vi "MCL Single Read N.vi"(8 "error in (no error)":errorcluster, 10 "handle":i32, 11 "axis":u32) -> (0 "error out":errorcluster, 3 "function return":dbl)   [LabVIEW 2014, in "Madlib.lvlib"]
doc: "MADLIB_API double MCL_SingleReadN(unsigned int axis, int handle);"
uses:
  <userlib>/Lambda2/lib/Madlib/Madlib.lvlib
  <userlib>/Lambda2/lib/Madlib/Madlib.dll
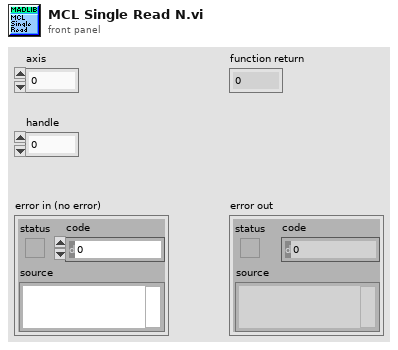
[diagram p1: front panel]
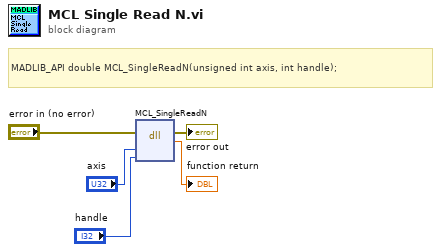
[diagram p0: block diagram]
diagram:
  # "MADLIB_API\tdouble\tMCL_SingleReadN(unsigned int axis, int handle);"
  n1 = dll-call lib="C:/Program Files (x86)/National Instruments/LabVIEW 2014/user.lib/Lambda2/lib/Madlib/Madlib.*" fn="MCL_SingleReadN"(error in="error in (no error)", "axis"="axis", "handle"="handle") -> (error out=→"error out":errorcluster, →"function return":dbl)  [unwired: 4 in, 1 out]
